vi "河内塔-子VI.vi"(3 "C":string, 4 "B":string, 5 "A":string, 6 "n":u8) -> ()   [LabVIEW 2016]
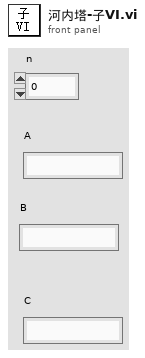
[diagram p1: front panel]
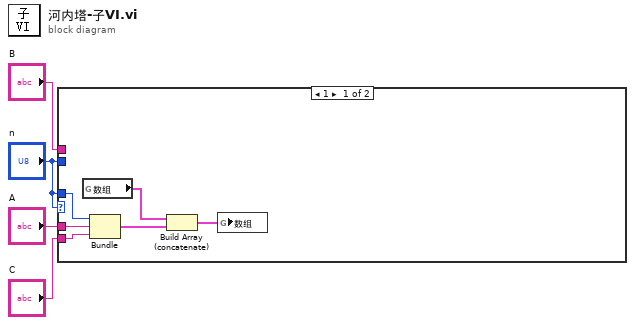
[diagram p0: block diagram]
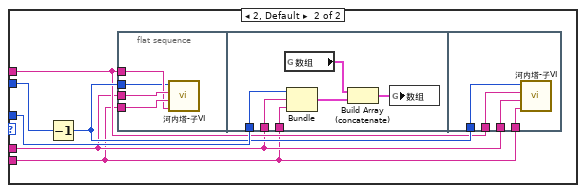
[diagram p2: hidden frame]
diagram:
  n1 = case shown="1" "n" {
    tunnel: "n" -> [w9 w16]
    tunnel: "A" -> [w8 w12]
    tunnel: "C" -> [w7 w11]
    tunnel: "n" -> [_ w15]
    tunnel: "B" -> [_ w13]
    frame 1 {
      n2 = global read "河内塔-全局.vi" "数组"() -> (w5:cluster{"n":u8, "From":string, "To":string}[])
      n3 = Bundle("n"=w9, "A"=w8, "C"=w7) -> (w10:cluster{"n":u8, "A":string, "C":string})  [unwired: 1 in]
      n4 = Build Array (concatenate)(w5, w10) -> (w6:cluster{"n":u8, "A":string, "C":string}[])
      n5 = global write "河内塔-全局.vi" "数组"(w6) -> ()
    }
    frame 2, Default {
      n6 = Decrement(x=w15) -> (x-1=w14:u8)
      n7 = flat-sequence {
        tunnel: w12 -> [w20]
        tunnel: w11 -> [w19]
        tunnel: w13 -> [w18]
        tunnel: w14 -> [w17]
        tunnel: w16 -> [w25]
        tunnel: w12 -> [w24]
        tunnel: w11 -> [w23]
        tunnel: w14 -> [w30]
        tunnel: w13 -> [w29]
        tunnel: w12 -> [w28]
        tunnel: w11 -> [w27]
        frame #0 {
          n8 = call "河内塔-子VI.vi"("C"=w18, "B"=w19, "A"=w20, "n"=w17) -> ()  [unwired: 3 in]
        }
        frame #1 {
          n9 = global read "河内塔-全局.vi" "数组"() -> (w21:cluster{"n":u8, "From":string, "To":string}[])
          n10 = Bundle("n"=w25, "A"=w24, "C"=w23) -> (w26:cluster{"n":u8, "A":string, "C":string})  [unwired: 1 in]
          n11 = Build Array (concatenate)(w21, w26) -> (w22:cluster{"n":u8, "A":string, "C":string}[])
          n12 = global write "河内塔-全局.vi" "数组"(w22) -> ()
        }
        frame #2 {
          n13 = call "河内塔-子VI.vi"("C"=w27, "B"=w28, "A"=w29, "n"=w30) -> ()  [unwired: 3 in]
        }
      }
    }
  }
